vi "1886_FGlob_CAN_Read.vi"(5 "Function (Recall One)":T1=enum."Recall one", 7 "CAN Read Items":u16=20, 8 "err in":errorcluster caption="error", 10 "AI Values IN":dbl[](array[numeric]) format="%.6f", 11 "AI Value IN":dbl format="%.6f") -> (0 "err out":errorcluster caption="error", 2 "AI Values OUT":dbl[](array[numeric]) format="%.6f", 3 "AI Value OUT":dbl format="%.6f")   [LabVIEW 2021]
uses:
  1886_FGlob_TDefs_Enum_FGlobItems.ctl
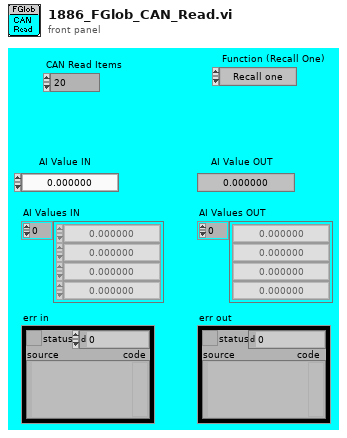
[diagram p1: front panel]
types:
  T1 = typedef "1886_FGlob_TDefs_Enum_FGlobItems.ctl" = enum16{"Put one", "Put all", "Recall one", "Recall all"}
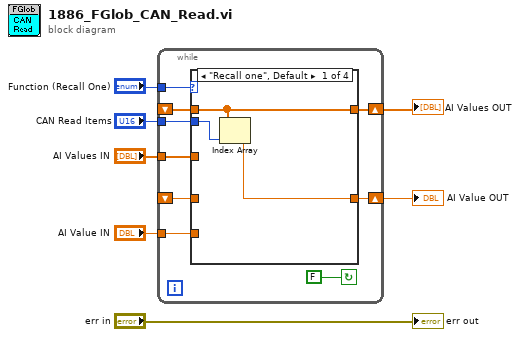
[diagram p0: block diagram]
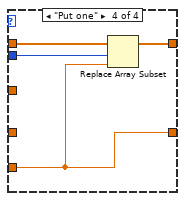
[diagram p4: hidden frame]
diagram:
  n1 = while {
    shift-right: [w14] -> w5
    shift-left: _ -> [w13]
    tunnel: "Function (Recall One)" -> [w15]
    tunnel: "CAN Read Items" -> [w11]
    tunnel: "AI Values IN" -> [w10]
    shift-right: [w12] -> w4
    shift-left: _ -> [w9]
    tunnel: "AI Value IN" -> [w8]
    stop <- FALSE continue-if-true
    n2 = case shown="\"Recall one\", Default" w15 {
      tunnel: [w19 w21 w23 w26] -> w14
      tunnel: w13 -> [w19 w21 _ w27]
      tunnel: w11 -> [w17 _ _ w25]
      tunnel: [w18 w20 w22 w24] -> w12
      tunnel: w10 -> [_ _ w23 _]
      tunnel: w9 -> [_ w20 w22 _]
      tunnel: w8 -> [_ _ _ w24]
      frame "Recall one", Default {
        n3 = Index Array(array=w19, index=w17) -> (element=w18:dbl)
      }
      frame "Recall all" {
      }
      frame "Put all" {
      }
      frame "Put one" {
        n4 = Replace Array Subset(array=w27, new element=w24, index=w25) -> (w26:dbl[])
      }
    }
  }
  "AI Values OUT" <- w5
  "AI Value OUT" <- w4
  "err out" <- "err in"
